vi "_Remote BlockUpdate.vi"(4 "error in":errorcluster, 6 "Filter (T)":bool=TRUE, 7 "Running":bool) -> (0 "error out":errorcluster)   [LabVIEW 2015]
uses:
  Type/_RT Active Ch.ctl
  Type/_RT Command.ctl
  Configuration/_Global Configuration.vi
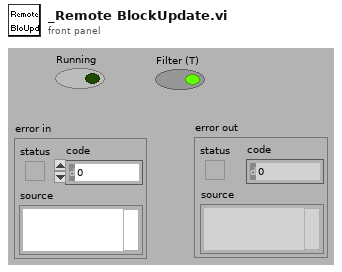
[diagram p1: front panel]
types:
  T1 = typedef "_RT Active Ch.ctl" = cluster{"Start":i32, "Step":i32, "ChID":i32}
  T2 = typedef "_Lens Property.ctl" = cluster{"Scan Type":u8, "Scans":i32, "Time 1":dbl, "Time 2":dbl, "Value 1":dbl, "Value 2":dbl, "Step Size":dbl}
  T3 = typedef "_Mass Range Property.ctl" = cluster{"Start":dbl, "Stop":dbl, "Step Size":dbl, "Steps":i32, "Dwell":dbl, "Parameters":T4[], "Res":T5}
  T4 = typedef "_Mass Range Parameters.ctl" = cluster{"Name":string, "Ch#":u8, "StartV":dbl, "StopV":dbl, "StepV":dbl, "Index":u8}
  T5 = typedef "_RT Res Type.ctl" = u16
  T6 = typedef "_Run Mode.ctl" = enum16{"MRM (Q1/Q2)", "Q1 Scan", "Q1 SRM", "Q2 Scan", "Q2 SRM", "Product Scan", "Precursor Scan", "Neutral Loss", "Neutral Gain"}
  T7 = cluster{"Lenses":T2[], "Mass Ranges":T3[], "Acquire":bool, "MCA":bool, "Q1DC EN":bool, "Q1 POL":bool, "Q3 POL":bool, "Q1 RF  EN":bool, "Averaging":bool, "Log Scale":bool, "CPS":bool, "Unit":bool, "Data Path":path, "Run Mode":T6, "Fixed Mass (amu)":dbl, "Q3DC EN":bool, "Q3 RF  EN":bool, "Negative":bool}
  T8 = typedef "_RT Instrument 2.ctl" = cluster{"Table":T9[], "Instrument":string[]}
  T9 = typedef "_RT Configuration 2.ctl" = cluster{"Name":string, "Ch#":u8, "Min":dbl, "Max":dbl, "Def+":dbl, "Def-":dbl, "Offset":dbl, "Slope":dbl, "Type":u8, "Description":string, "SettleT":dbl}
  T10 = typedef "_RT Command.ctl" = enum16{"xml Start Run", "xml Start Actual Run", "xml Stop Run", "xml Runtime Update", "xml Get Status", "xml Get Table", "xml Set Table", "xml Get Configuration", "xml System Status", "xml Set LC Input Logic", "xml Get Data", "xml Get Info", "Start", "StartActualRun", "Stop", "Runtime Update", "Get Data", "Get Info", "Get Status", "Get Param", "Get Config", "Get Table", "Read ADC", "Set Oscillator", "Update Config", "Update Table", "Set All Pol", "Set Pol and DC", "Set Max Mass", "Toggle RP", "Toggle EL", "Set PIC", "Initialize Turbo", "Send Turbo Comm", "Close Turbo", "P1", "P2", "P3", "Send Serial", "Set LC Out", "Get LC In", "Read VAC", "Test Table", "Toggle Power", "Get Startup", "Set Startup", "Get ADC Table", "Set ADC Table", "Get Brief Status", "Get Detail Status", "Auxiliary Update", "Set CC Logics", "Set CC Input Logics", "Ignore Error", "invalid"}
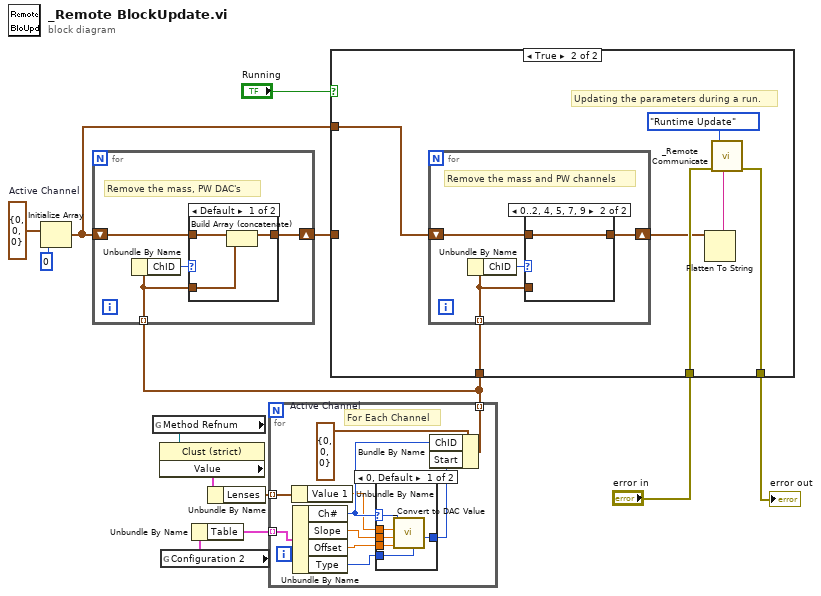
[diagram p0: block diagram]
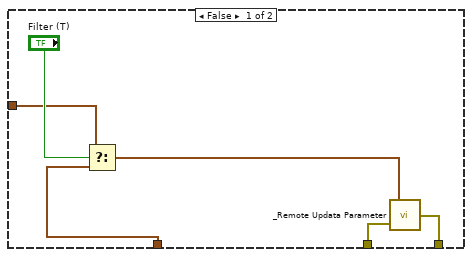
[diagram p3: hidden frame]
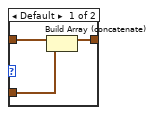
[diagram p4: hidden frame]
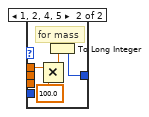
[diagram p5: hidden frame]
diagram:
  w4 = T1 {"Start"=0, "Step"=0, "ChID"=0}  # Active Channel
  n1 = Initialize Array(w4, 0 ("dimension size")) -> (w1:T1[])
  n2 = global read "_Global Configuration.vi" "Method Refnum"() -> (w10:refnum<vi>)
  n3 = property class="Clust (strict)"(reference=w10) -> ("Value"=w8:T7)  [unwired: 1 in, 2 out]
  n4 = global read "_Global Configuration.vi" "Configuration 2"() -> (w9:T8)
  n5 = Unbundle By Name(w9) -> ("Table"=w11:T9[])
  n6 = Unbundle By Name(w8) -> ("Lenses"=w7:T2[])
  n7 = for {
    tunnel: [w19] -> w3 mode=indexing
    tunnel: w11 -> [w17] mode=indexing
    tunnel: w7 -> [w16] mode=indexing
    w21 = T1 {"Start"=0, "Step"=0, "ChID"=0}  # Active Channel
    # "For Each Channel"
    n8 = Unbundle By Name(w16) -> ("Value 1"=w15:dbl)
    n9 = Unbundle By Name(w17) -> ("Ch#"=w18:u8, "Slope"=w23:dbl, "Offset"=w22:dbl, "Type"=w14:u8)
    n10 = case shown="0, Default" w18 {
      selector: w18 -> [w25 _]
      tunnel: w15 -> [w29 w33]
      tunnel: w23 -> [w28 _]
      tunnel: w22 -> [w27 _]
      tunnel: [w26 w30] -> w20
      tunnel: w14 -> [w24 _]
      frame 0, Default {
        n11 = call "_Convert to DAC Value.vi"("Type"=w24, "Offset"=w27, "Slop"=w28, "Number"=w29, "Channel"=w25) -> ("DAC Value"=w26:i32)  [unwired: 2 in, 4 out]
      }
      frame 1, 2, 4, 5 {
        # "for mass"
        n12 = Multiply(x=w33, y=100.0) -> (x*y=w31:dbl)
        n13 = To Long Integer(number=w31) -> (32bit integer=w30:i32)
      }
    }
    n14 = Bundle By Name(cluster=w21, "ChID"=w18, "Start"=w20) -> (w19:T1)
  }
  n15 = for {
    shift-right: [w35] -> w2
    shift-left: w1 -> [w36]
    tunnel: w3 -> [w34] mode=indexing
    # "Remove the mass, PW DAC's"
    n16 = Unbundle By Name(w34) -> ("ChID"=w37:i32)
    n17 = case shown="Default" w37 {
      tunnel: [w38 w41] -> w35
      tunnel: w36 -> [w40 w41]
      tunnel: w34 -> [w39 _]
      frame Default {
        n18 = Build Array (concatenate)(w40, w39) -> (w38:T1[])
      }
      frame 0..2, 4, 5, 7, 9 {
      }
    }
  }
  n19 = case shown="True" "Running" {
    tunnel: "error in" -> [w43 w53]
    tunnel: [w44 w52] -> w12
    tunnel: w3 -> [w45 w50]
    tunnel: w2 -> [w46 _]
    tunnel: w1 -> [_ w48]
    frame False {
      n20 = Select(t=w46, s="Filter (T)", f=w45) -> (s? t:f=w42:T1[])
      n21 = call "_Remote Updata Parameter.vi"("error in"=w43, "Parameters"=w42) -> ("error out"=w44:errorcluster)
    }
    frame True {
      # "Updating the parameters during a run."
      n22 = for {
        shift-right: [w56] -> w49
        shift-left: w48 -> [w57]
        tunnel: w50 -> [w55] mode=indexing
        # "Remove the mass and PW channels"
        n23 = Unbundle By Name(w55) -> ("ChID"=w58:i32)
        n24 = case shown="0..2, 4, 5, 7, 9" w58 {
          tunnel: [w59 w62] -> w56
          tunnel: w57 -> [w61 w62]
          tunnel: w55 -> [w60 _]
          frame Default {
            n25 = Build Array (concatenate)(w61, w60) -> (w59:T1[])
          }
          frame 0..2, 4, 5, 7, 9 {
          }
        }
      }
      n26 = Flatten To String(anything=w49) -> (data string=w51:string)  [unwired: 1 in, 4 out]
      n27 = call "_Remote Communicate.vi"("String"=w51, "error in (no error)"=w53, "Command"=_RT_Command."Runtime Update") -> ("error out"=w52:errorcluster)  [unwired: 3 in, 3 out]
    }
  }
  "error out" <- w12
